vi "Active Noise Control with Feedback Neutralization (FPGA).vi"() -> ()   [LabVIEW 2019]
doc: "This VI runs on an FPGA target. \nFirstly, this VI generates a stimulus waveform for the control speaker and acquires waveforms through the error microphone and primary microphone for feedback path and secondary path modeling.\nSecondly, this VI retrieves the coefficients of the feedback path and secondary path. \nFinally, this VI uses a filtered-X LMS adaptive filter to generate a control waveform for the control speaker."
uses:
  <vilib>/LabVIEW Targets/FPGA/cRIO/shared/nicrio_ModuleControls/nicrio_cRIO-9233_DataRatesRing.ctl
  <vilib>/rvi/eio/common/nirviEmuTemplatePropertySet_noerrors.vi
  <vilib>/rvi/eio/common/nirviEmuTemplateMethod_errors.vi
  <vilib>/rvi/Emulation/niFpgaGetClockAttributes.vi
  <vilib>/rvi/Emulation/niFpgaSctlEmulationGetInTimedLoop.vi
  <vilib>/rvi/Emulation/niFpgaEmulationReportErrorSimple.vi
  <vilib>/rvi/interface/RandomDataEmulation/niFpgaRandomDataHandleErrors.vi
  <vilib>/rvi/Emulation/niFpgaCriticalErrorInLSC.vi
  <vilib>/rvi/Memory/Memory_Emulation/nirvimemoryEmulation.vi
  <vilib>/rvi/Memory/Memory_Emulation/nirvimemoryFastEmulation.vi
  <vilib>/rvi/DataTransferAndStorage/Container/Common/niFpgaContainerGetUniqueNameForEmu.vi
  <vilib>/rvi/Memory/Memory_Emulation/niFpgaMemoryEmulationCacheClearOnFirstRun.vi
  <vilib>/rvi/Memory/Memory_Emulation/nirvimemoryEmulationManagerCache_MakeExclusive.vi
  <vilib>/rvi/Memory/Memory_Emulation/niFpgaMemoryEmulationValidateCache.vi
  <vilib>/rvi/Memory/Memory_Emulation/nirvimemoryEmulationManagerCache_InsertValue.vi
  <vilib>/Utility/error.llb/Clear Errors.vi
  <vilib>/rvi/Memory/Memory_Emulation/nirvimemoryEmulationManagerCache_ReleaseExclusive.vi
  <vilib>/rvi/Memory/Memory_Emulation/nirvimemoryEmulationManagerCache_GetValue.vi
  <vilib>/rvi/Emulation/niFpgaEmulationIsFPGAContextNoSignature.vi
  <vilib>/rvi/Memory/Memory_Emulation/nirvimemoryEmulationManagerCache_SetValue.vi
  <vilib>/rvi/Emulation/niFpgaSctlEmulationResourceMgr.vi
  <vilib>/eio/EIOPropertyNode/EIOPropertyNode.xnode
  <vilib>/LabVIEW Targets/FPGA/cRIO/shared/nicrio_ModuleControls/nicrio_cRIO-9234_DataRatesRing2.ctl
  <vilib>/eio/EIONode/EIONode.xnode
  <vilib>/rvi/DataTransferAndStorage/Container/XNode/niFpgaContainer.xnode
  <vilib>/rvi/interface/RandomDataEmulation/nirviRandomDataFpgaReadWriteTemplate.vi
  <vilib>/rvi/eio/common/nirviEmuTemplatePropertyGet_errors.vi
  <vilib>/rvi/eio/common/nirviEmuTemplatePropertyGet_noerrors.vi
  <vilib>/rvi/eio/common/nirviEmuTemplatePropertySet_errors.vi
panel:
  in  "stop modeling":bool
  in  "filter length":u32
  in  "control on":bool
  in  "reset? (F)":bool
  in  "step size":fxp<+/-,16,-2>
  in  "stop":bool
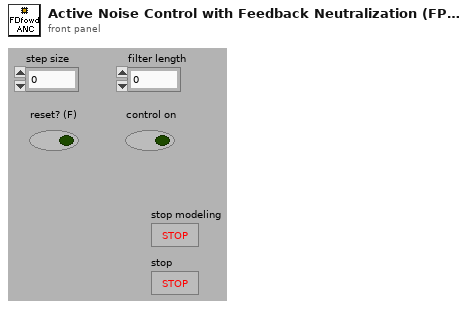
[diagram p1: front panel]
types:
  T1 = typedef "nicrio_cRIO-9233_DataRatesRing.ctl" = u8
  T2 = cluster{"x(n)":fxp<+/-,32,4>, "fx(n)":fxp<+/-,32,4>, "y(n)":fxp<+/-,32,4>}
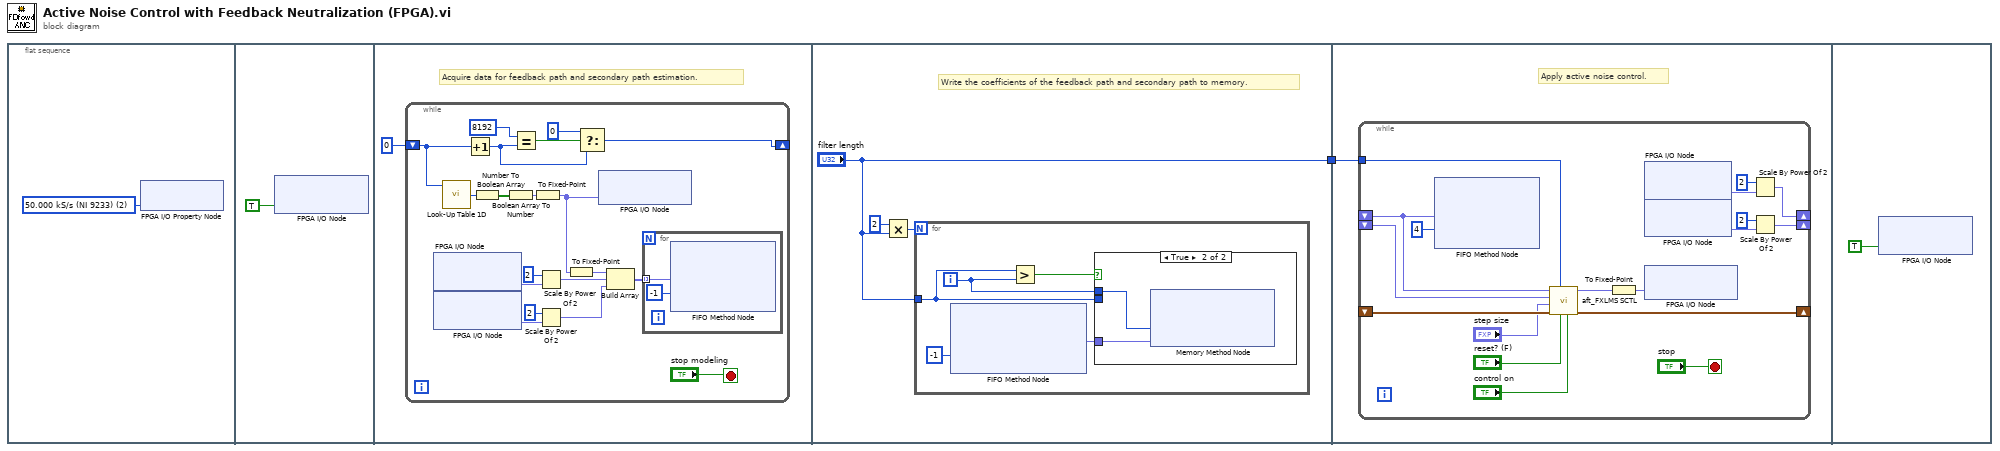
[diagram p0: block diagram]
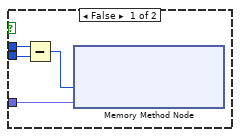
[diagram p2: hidden frame]
diagram:
  n1 = flat-sequence {
    tunnel: ["filter length"] -> w1
    tunnel: w1 -> [w40]
    frame #0 {
      w2 = T1 2 items=["50.000 kS/s (NI 9233)"=2, "33.333 kS/s (NI 9233)"=3, "25.000 kS/s (NI 9233)"=34, "16.667 kS/s (NI 9233)"=35, "12.500 kS/s (NI 9233)"=36, "10.000 kS/s (NI 9233)"=37, "  8.333 kS/s (NI 9233)"=38, "  7.143 kS/s (NI 9233)"=39, "  6.250 kS/s (NI 9233)"=40, "  5.556 kS/s (NI 9233)"=41, "  5.000 kS/s (NI 9233)"=42, "  4.545 kS/s (NI 9233)"=43, "  4.167 kS/s (NI 9233)"=44, "  3.846 kS/s (NI 9233)"=45, "  3.571 kS/s (NI 9233)"=46, "  3.333 kS/s (NI 9233)"=47, "  3.125 kS/s (NI 9233)"=48, "  2.941 kS/s (NI 9233)"=49, "  2.778 kS/s (NI 9233)"=50, "  2.632 kS/s (NI 9233)"=51, "  2.500 kS/s (NI 9233)"=52, "  2.381 kS/s (NI 9233)"=53, "  2.273 kS/s (NI 9233)"=54, "  2.174 kS/s (NI 9233)"=55, "  2.083 kS/s (NI 9233)"=56, "  2.000 kS/s (NI 9233)"=57] ("Data Rate")
      n2 = xnode "FPGA I/O Property Node"("Data Rate"=w2) -> ()  [unwired: 1 in, 1 out]
    }
    frame #1 {
      n3 = xnode "FPGA I/O Node"("Mod1/Start"=TRUE) -> ()  [unwired: 2 in, 2 out]
    }
    frame #2 {
      # "Acquire data for feedback path and secondary path estimation."
      n4 = while {
        shift-right: [w5] -> _
        shift-left: u16 0 -> [w7]
        stop <- "stop modeling" stop-if-true
        n5 = xnode "FPGA I/O Node"() -> ("Mod1/AI1"=w22:fxp<+/-,24,4>)  [unwired: 2 in, 2 out]
        n6 = xnode "FPGA I/O Node"() -> ("Mod1/AI0"=w23:fxp<+/-,24,4>)  [unwired: 2 in, 2 out]
        n7 = call "Look-Up Table 1D"("address"=w7) -> ("data out"=w10:i16)  [unwired: 8 in]
        n8 = Increment(x=w7) -> (x+1=w14:u16)
        n9 = Number To Boolean Array(number=w10) -> (Boolean array=w11:bool[])
        n10 = Boolean Array To Number(Boolean array=w11) -> (number=w12:fxp<+/-,16,1>)
        n11 = Equal?(x=u16 8192 ("y"), y=w14) -> (x = y?=w8:bool)
        n12 = To Fixed-Point(number=w12) -> (fixed-point=w6:fxp<+/-,20,5>)  [unwired: 1 out]
        n13 = Scale By Power Of 2(n=2 ("gain for microphone channel"), x=w22) -> (x*2^n=w16:fxp<+/-,24,4>)
        n14 = Scale By Power Of 2(n=2 ("gain for microphone channel"), x=w23) -> (x*2^n=w15:fxp<+/-,24,4>)
        n15 = To Fixed-Point(number=w6) -> (fixed-point=w21:fxp<+/-,24,4>)  [unwired: 1 in]
        n16 = Select(t=u16 0, s=w8, f=w14) -> (s? t:f=w5:u16)
        n17 = xnode "FPGA I/O Node"("Mod2/AO0"=w6) -> ()  [unwired: 1 in, 1 out]
        n18 = Build Array(w21, w16, w15) -> (w20:fxp<+/-,24,4>[])
        n19 = for {
          tunnel: w20 -> [w25] mode=indexing
          n20 = xnode ("FIFO Method Node")("Element"=w25, "Timeout"=-1) -> ()  [unwired: 1 in, 2 out]
        }
      }
    }
    frame #3 {
      # "Write the coefficients of the feedback path and secondary path to memory."
      n21 = Multiply(x=u32 2 ("y"), y="filter length") -> (x*y=w28:u32)
      n22 = for {
        N: w28 -> [_]
        tunnel: "filter length" -> [w29]
        i -> [w31]
        n23 = xnode ("FIFO Method Node")("Timeout"=-1) -> ("Element"=w33:fxp<+/-,32,4>)  [unwired: 1 in, 2 out]
        n24 = Greater?(x=w29, y=w31) -> (0:w30:bool)
        n25 = case shown="True" w30 {
          tunnel: w33 -> [w37 w39]
          tunnel: w31 -> [w36 w38]
          tunnel: w29 -> [w35 _]
          frame False {
            n26 = Subtract(x=w36, y=w35) -> (x-y=w34:u32)
            n27 = xnode ("Memory Method Node")("Address"=w34, "Data"=w37) -> ()  [unwired: 1 in, 1 out]
          }
          frame True {
            n28 = xnode ("Memory Method Node")("Address"=w38, "Data"=w39) -> ()  [unwired: 1 in, 1 out]
          }
        }
      }
    }
    frame #4 {
      # "Apply active noise control."
      n29 = while {
        shift-right: [w57] -> _
        shift-left: _ -> [w56]
        shift-right: [w55] -> _
        shift-left: _ -> [w45]
        shift-right: [w53] -> _
        shift-left: _ -> [w42]
        tunnel: w40 -> [w51]
        stop <- "stop" stop-if-true
        n30 = xnode ("FIFO Method Node")("Element"=w42, "Timeout"=4) -> ()  [unwired: 1 in, 2 out]
        n31 = call "aft_FXLMS SCTL.vi"("control on"="control on", "reset? (F)"="reset? (F)", "filter length"=w51, "status in"=w56, "step size"="step size", "ref mic"=w45, "error mic"=w42) -> ("status out"=w57:T2, "y(n)"=w46:fxp<+/-,24,4>)  [unwired: 3 in]
        n32 = To Fixed-Point(number=w46) -> (fixed-point=w47:fxp<+/-,20,5>)  [unwired: 1 in]
        n33 = xnode "FPGA I/O Node"() -> ("Mod1/AI0"=w52:fxp<+/-,24,4>)  [unwired: 2 in, 2 out]
        n34 = xnode "FPGA I/O Node"() -> ("Mod1/AI1"=w54:fxp<+/-,24,4>)  [unwired: 2 in, 2 out]
        n35 = xnode "FPGA I/O Node"("Mod2/AO0"=w47) -> ()  [unwired: 1 in, 1 out]
        n36 = Scale By Power Of 2(n=2, x=w52) -> (x*2^n=w53:fxp<+/-,24,4>)
        n37 = Scale By Power Of 2(n=2, x=w54) -> (x*2^n=w55:fxp<+/-,24,4>)
      }
    }
    frame #5 {
      n38 = xnode "FPGA I/O Node"("Mod1/Stop"=TRUE) -> ()  [unwired: 2 in, 2 out]
    }
  }
